vi "AddInstance.vi"(8 "error in (no error)":errorcluster, 11 "RQMHLogger in":refnum<class "Logger.lvclass">) -> (0 "error out":errorcluster)   [LabVIEW 2024, in "LogSingleton.lvlib"]
uses:
  LogSingleton.lvlib
  RQMHLogger/Logger.lvclass
  RQMHLogger/Logger.lvclass/Logger.ctl
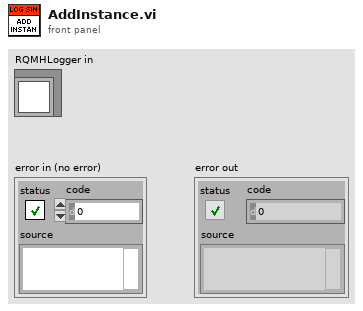
[diagram p1: front panel]
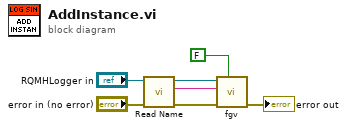
[diagram p0: block diagram]
diagram:
  n1 = call "Read Name.vi"("error in (no error)"="error in (no error)", "RQMHLogger in"="RQMHLogger in") -> ("error out"=w3:errorcluster, "Name"=w5:string, "RQMHLogger out"=w6:refnum<class "Logger.lvclass">)  [unwired: 7 in]
  n2 = call "fgv.vi"("Get? (T)"=FALSE, "error in (no error)"=w3, "Logger Name"=w5, "RQMHLogger Set"=w6) -> ("error out"=→"error out":errorcluster)  [unwired: 6 in, 1 out]
